vi "获取昨天日期.vi"() -> (3 "FROM:":string)   [LabVIEW 2017]
panel:
  in  "日期格式":string="/"
  out "昨天日期":string
  out "日":string
  out "月":string
  out "年":string
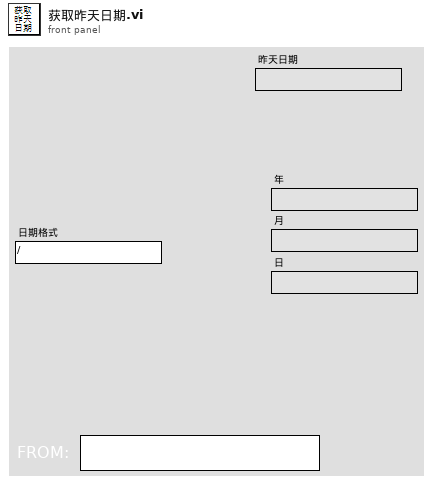
[diagram p1: front panel]
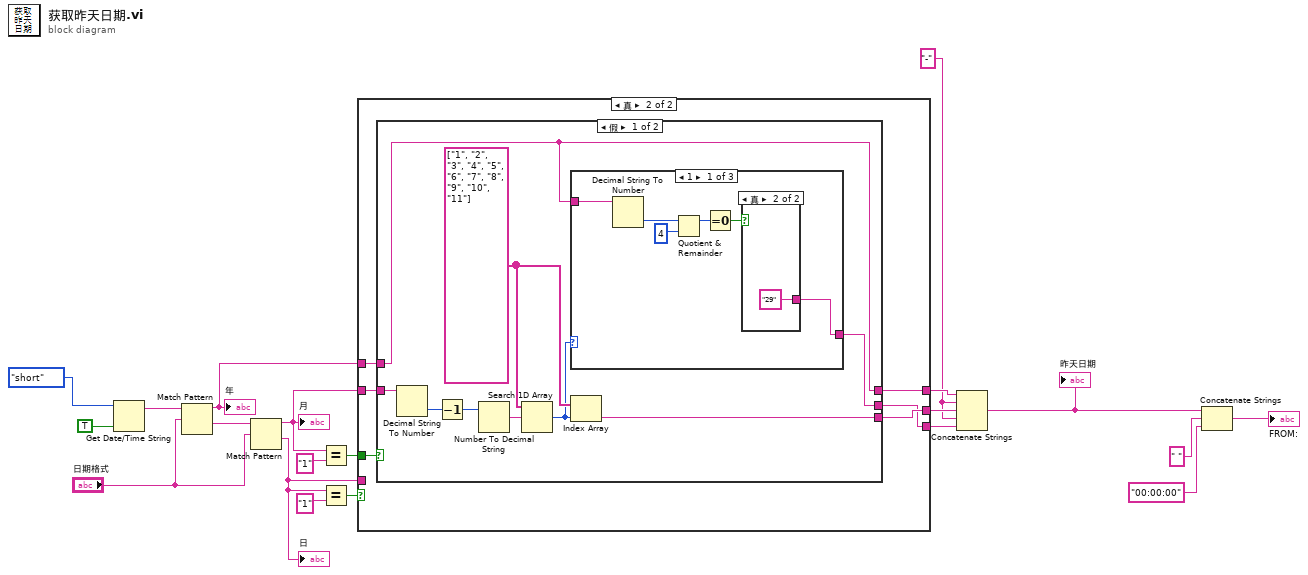
[diagram p0: block diagram]
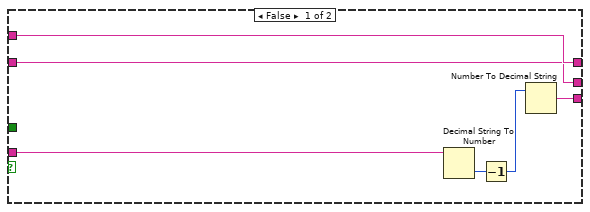
[diagram p2: hidden frame]
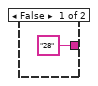
[diagram p3: hidden frame]
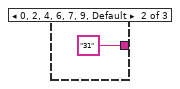
[diagram p4: hidden frame]
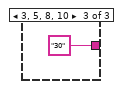
[diagram p5: hidden frame]
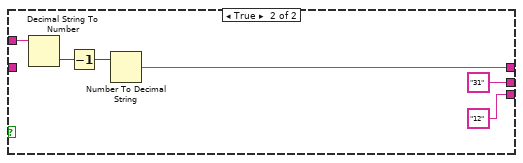
[diagram p6: hidden frame]
diagram:
  w7 = "-" ("正则表达式")
  n1 = Get Date/Time String(date format (0)=enum16{"short", "long", "abbreviated"}."short" ("日期格式(0)"), want seconds? (F)=TRUE ("需要秒？(F)")) -> (date string=w16:string)  [unwired: 1 in, 1 out]
  n2 = Match Pattern(string=w16, regular expression="日期格式") -> (before substring=w10:string, after substring=w15:string)  [unwired: 1 in, 2 out]
  "年" <- w10
  n3 = Match Pattern(string=w15, regular expression="日期格式") -> (before substring=w5:string, after substring=w4:string)  [unwired: 1 in, 2 out]
  "月" <- w5
  "日" <- w4
  n4 = Equal?(x=w5, y="1") -> (x = y?=w11:bool)
  n5 = Equal?(x=w4, y="1") -> (x = y?=w12:bool)
  n6 = case shown="真" w12 {
    tunnel: w11 -> [_ w32]
    tunnel: w10 -> [w22 w31]
    tunnel: [w22 w30] -> w9
    tunnel: [w21 w29] -> w8
    tunnel: [w23 w28] -> w6
    tunnel: w5 -> [w21 w27]
    tunnel: w4 -> [w24 _]
    frame False {
      n7 = Decimal String To Number(string=w24) -> (number=w26:i32)  [unwired: 2 in, 1 out]
      n8 = Decrement(x=w26) -> (x-1=w25:i32)
      n9 = Number To Decimal String(number=w25) -> (decimal integer string=w23:string)  [unwired: 1 in]
    }
    frame True {
      n10 = case shown="假" w32 {
        tunnel: w31 -> [w37 w56]
        tunnel: [w37 w54] -> w30
        tunnel: [w38 "12" ("正则表达式")] -> w29
        tunnel: [w41 "31" ("正则表达式")] -> w28
        tunnel: w27 -> [w34 _]
        frame False {
          w40 = string[] ["1", "2", "3", "4", "5", "6", "7", "8", "9", "10", "11"] ("一维数组")
          n11 = Decimal String To Number(string=w34) -> (number=w35:i32)  [unwired: 2 in, 1 out]
          n12 = Decrement(x=w35) -> (x-1=w36:i32)
          n13 = Number To Decimal String(number=w36) -> (decimal integer string=w33:string)  [unwired: 1 in]
          n14 = Search 1D Array(1D array=w40, element=w33) -> (index of element=w39:i32)  [unwired: 1 in]
          n15 = case shown="1" w39 {
            tunnel: [w42 "31" "30"] -> w41
            tunnel: w37 -> [w43 _ _]
            frame 1 {
              n16 = Decimal String To Number(string=w43) -> (number=w44:i32)  [unwired: 2 in, 1 out]
              n17 = Quotient & Remainder(x=w44, y=4) -> (x-y*floor(x/y)=w46:i32)  [unwired: 1 out]
              n18 = Equal To 0?(x=w46) -> (x = 0?=w47:bool)
              n19 = case shown="真" w47 {
                tunnel: ["28" "29"] -> w42
                frame False {
                }
                frame True {
                }
              }
            }
            frame 0, 2, 4, 6, 7, 9, Default {
            }
            frame 3, 5, 8, 10 {
            }
          }
          n20 = Index Array(array=w40, index=w39) -> (element=w38:string)
        }
        frame True {
          n21 = Decimal String To Number(string=w56) -> (number=w55:i32)  [unwired: 2 in, 1 out]
          n22 = Decrement(x=w55) -> (x-1=w57:i32)
          n23 = Number To Decimal String(number=w57) -> (decimal integer string=w54:string)  [unwired: 1 in]
        }
      }
    }
  }
  n24 = Concatenate Strings(w9, w7, w8, w7, w6) -> (w3:string)
  "昨天日期" <- w3
  n25 = Concatenate Strings(w3, " " ("字符串"), "00:00:00" ("字符串")) -> (→"FROM:":string)
